vi "Create.vi"(8 "error in (no error)":errorcluster) -> (0 "error out":errorcluster, 3 "Result Model out":refnum<class "Result Model.lvclass">)   [LabVIEW 2020, in "Result Model.lvclass"]
uses:
  Result Model/Result Model.lvclass
  Result Model/Result Model.lvclass/Result Model.ctl
  Core/Result/Status.ctl
  Core/Result/Result.lvlib
  Core/Result/Type.ctl
  Core/Result/Result.ctl
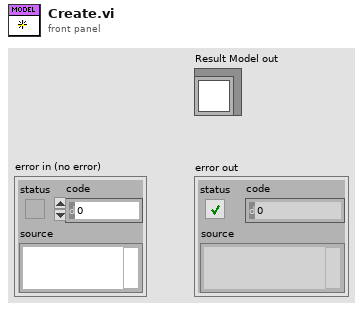
[diagram p1: front panel]
types:
  T1 = typedef "Result.lvlib/Status.ctl" = enum16{"", "Passed", "Failed", "Error", "Skipped", "Setup Error", "Broken", "Teardown Error"}
  T2 = typedef "Result.lvlib/Type.ctl" = enum16{"Test Case", "Test Suite", "Test Run", "Pass", "Fail", "Skip", "Pass if", "Fail if", "Pass if Error", "Fail if Error", "Pass if Equal", "Fail if Equal"}
  T3 = cluster{"Tests":string[], "Run Queue":string[], "Test Statuses":map{string, T1}, "Execution Time":map{string, dbl}, "Assertions":map{string, cluster{"Result Type":T2, "Status":T1, "Description":string, "Data":cluster{"Expected":variant, "Actual":variant, "Delta":variant}}[]}}
  T4 = typedef "Result.lvlib/Result.ctl" = cluster{"Name":string, "Description":string, "Status":T1, "Result Type":T2, "Execution Time":dbl, "Data":cluster{"Expected":variant, "Actual":variant, "Delta":variant}}
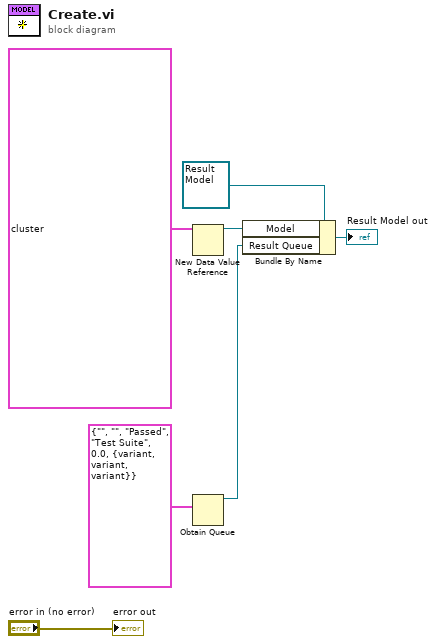
[diagram p0: block diagram]
diagram:
  n1 = New Data Value Reference(data value=T3 {"Tests"=[], "Run Queue"=[], "Test Statuses"={}, "Execution Time"={}, "Assertions"={}} ("Cluster of class private data")) -> (data value reference=w1:refnum<data-value>)  [unwired: 1 in, 1 out]
  n2 = Obtain Queue(element data type=T4 {"Name"="", "Description"="", "Status"=enum."Passed", "Result Type"=enum."Test Suite", "Execution Time"=0.0, "Data"={"Expected"=variant, "Actual"=variant, "Delta"=variant}} ("Results")) -> (queue out=w3:refnum<queue>)  [unwired: 4 in, 2 out]
  n3 = Bundle By Name(cluster=refnum<class "Result Model.lvclass"> refnum ("Result Model in"), "Model"=w1, "Result Queue"=w3) -> (→"Result Model out":refnum<class "Result Model.lvclass">)
  "error out" <- "error in (no error)"
